vi "TCP Create Arbitrary Listener.vi"(8 "error in (no error)":errorcluster, 10 "port (use next available)":u16, 11 "address (any)":string) -> (0 "error out":errorcluster, 2 "port used":u16, 3 "listener ID":refnum<k5>)   [LabVIEW 2020, in "NI_FTP.lvlib"]
doc: "Same as TCP Create Listener. When the port input is not connected, this VI uses the next available port (>= 1024). The allocated port is returned in the \"port used\" parameter."
uses:
  <vilib>/FTP/NI_FTP.lvlib
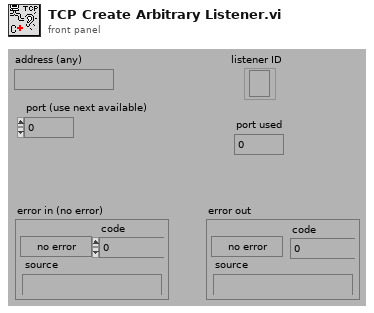
[diagram p1: front panel]
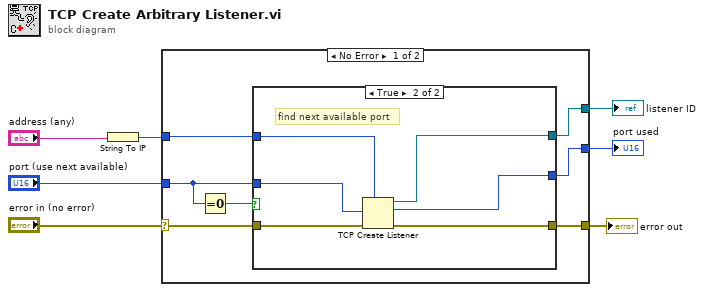
[diagram p0: block diagram]
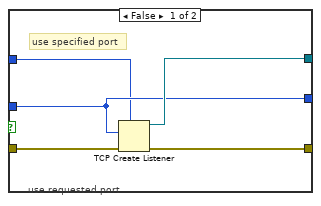
[diagram p2: hidden frame]
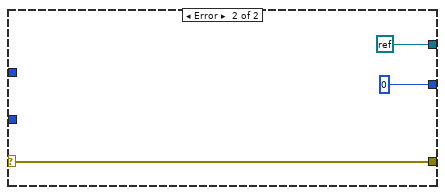
[diagram p3: hidden frame]
diagram:
  n1 = String To IP(1:"address (any)") -> (0:w1:u32)
  n2 = case shown="No Error" "error in (no error)" {
    selector: "error in (no error)" -> [w9 w26]
    tunnel: [w13 w26] -> w7
    tunnel: [w11 refnum<k0> refnum] -> w6
    tunnel: "port (use next available)" -> [w12 _]
    tunnel: [w10 u16 0] -> w4
    tunnel: w1 -> [w8 _]
    frame No Error {
      n3 = Equal To 0?(x=w12) -> (x = 0?=w14:bool)
      n4 = case shown="True" w14 {
        tunnel: w9 -> [w19 w25]
        tunnel: [w18 w24] -> w13
        tunnel: w12 -> [w16 w21]
        tunnel: [w17 w23] -> w11
        tunnel: [w16 w22] -> w10
        tunnel: w8 -> [w15 w20]
        frame False {
          # "use specified port"
          # "use requested port"
          n5 = TCP Create Listener(7:w15, 8:w19, 10:w16) -> (0:w18:errorcluster, 3:w17:refnum<k5>)  [unwired: 3 out]
        }
        frame True {
          # "find next available port"
          n6 = TCP Create Listener(7:w20, 8:w25, 10:w21) -> (0:w24:errorcluster, 2:w22:u16, 3:w23:refnum<k5>)  [unwired: 2 out]
        }
      }
    }
    frame Error {
    }
  }
  "listener ID" <- w6
  "error out" <- w7
  "port used" <- w4
